vi "stage track mode.vi"(8 "error in":errorcluster, 9 "speed":dbl, 10 "target":dbl, 11 "XPS Reference IN":refnum<k24>) -> (0 "error out":errorcluster, 3 "XPS Reference OUT":refnum<k24>)   [LabVIEW 2015]
uses:
  D:/labview program/whole brain TP_220607/sub vi/XPS-UNIFIED/LabVIEW VIs/LabVIEW Source Code/Dll/Newport.XPS.CommandInterface.dll
  XPS-UNIFIED/LabVIEW VIs/LabVIEW Source Code/Dll/Newport.XPS.CommandInterface.dll
  <vilib>/DAQmx/write.llb/DAQmx Write (Analog DBL 1Chan 1Samp).vi
  <vilib>/DAQmx/create/channels.llb/DAQmx Create Channel (AO-Voltage-Basic).vi
  <vilib>/DAQmx/miscellaneous.llb/DAQmx Fill In Error Info.vi
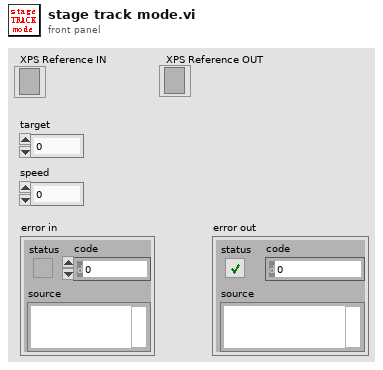
[diagram p1: front panel]
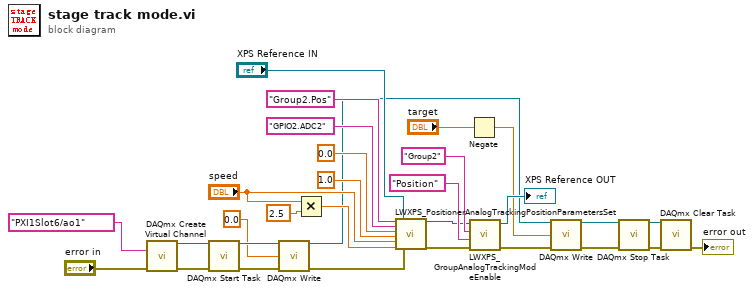
[diagram p0: block diagram]
diagram:
  n1 = call-poly <vilib>:"DAQmx Create Virtual Channel.vi"("physical channels"=tag "PXI1Slot6/ao1" ("Physical Channel(s)"), "error in"="error in") -> ("task out"=w17:refnum<k21>, "error out"=w16:errorcluster)  [unwired: 12 in]
  n2 = call <vilib>:"DAQmx Start Task.vi"("task/channels in"=w17, "error in"=w16) -> ("task out"=w15:refnum<k21>, "error out"=w14:errorcluster)  [unwired: 12 in]
  n3 = call-poly <vilib>:"DAQmx Write.vi"("task/channels in"=w15, "data"=0.0, "error in"=w14) -> ("task out"=w8:refnum<k21>, "error out"=w9:errorcluster)  [unwired: 10 in, 1 out]
  n4 = Multiply(x="speed", y=2.5) -> (x*y=w24:dbl)
  n5 = call "LWXPS_PositionerAnalogTrackingPositionParametersSet.vi"("Positioner Name"="Group2.Pos", "Analog input name"="GPIO2.ADC2", "Offset"=0.0 ("Offset1"), "Scale"=1.0 ("Scale1"), "Velocity"="speed", "Acceleration"=w24, "CommandInterfaceXPS.XPS"="XPS Reference IN", "LabVIEW error IN"=w9) -> ("CommandInterfaceXPS.XPS"=w20:refnum<k24>, "LabVIEW error OUT"=w19:errorcluster)  [unwired: 8 in, 2 out]
  n6 = Negate(x="target") -> (-x=w1:dbl)
  n7 = call "LWXPS_GroupAnalogTrackingModeEnable.vi"("LabVIEW error IN"=w19, "Tracking Type"="Position", "Group Name"="Group2", "CommandInterfaceXPS.XPS"=w20) -> ("LabVIEW error OUT"=w3:errorcluster, "CommandInterfaceXPS.XPS"=→"XPS Reference OUT":refnum<k24>)  [unwired: 2 in, 2 out]
  n8 = call-poly <vilib>:"DAQmx Write.vi"("task/channels in"=w8, "data"=w1, "error in"=w3) -> ("task out"=w7:refnum<k21>, "error out"=w4:errorcluster)  [unwired: 10 in, 1 out]
  n9 = call <vilib>:"DAQmx Stop Task.vi"("task/channels in"=w7, "error in"=w4) -> ("task out"=w6:refnum<k21>, "error out"=w10:errorcluster)  [unwired: 12 in]
  n10 = call <vilib>:"DAQmx Clear Task.vi"("task in"=w6, "error in"=w10) -> ("error out"=→"error out":errorcluster)  [unwired: 13 in]
